vi "FXP info.vi"(8 "error in (no error)":errorcluster, 11 "Variant":variant) -> (0 "error out":errorcluster, 3 "child strings":string[](array[string]))   [LabVIEW 2019, in "DSF Configuration Utility.lvlib"]
uses:
  DSF Configuration Utility.lvlib
  <vilib>/Utility/Data Type/NI_Data Type.lvlib
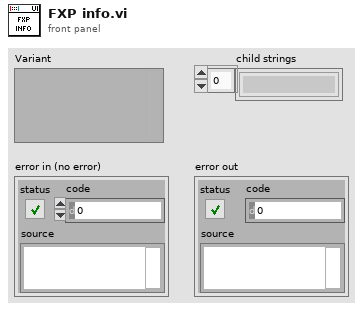
[diagram p1: front panel]
types:
  T1 = typedef "LVFixedPointRepRangeTypeDef.ctl" = cluster{"Range Min":dbl, "Range Max":dbl, "Delta":dbl}
  T2 = typedef "LVFixedPointRepBitsTypeDef.ctl" = cluster{"Signed":bool, "Word Length":u32, "Integer Word Length":i32}
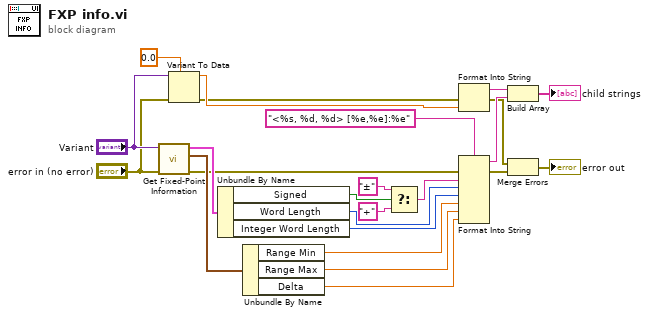
[diagram p0: block diagram]
diagram:
  n1 = call <vilib>:"Get Fixed-Point Information.vi"("error in (no error)"="error in (no error)", "variant"="Variant") -> ("error out"=w2:errorcluster, "FXP range"=w19:T1, "FXP representation"=w12:T2)  [unwired: 6 in, 1 out]
  n2 = Variant To Data(error in="error in (no error)", type=0.0, Variant="Variant") -> (data=w9:dbl, error out=w6:errorcluster)
  n3 = Unbundle By Name(w12) -> ("Signed"=w13:bool, "Word Length"=w17:u32, "Integer Word Length"=w18:i32)
  n4 = Unbundle By Name(w19) -> ("Range Min"=w20:dbl, "Range Max"=w21:dbl, "Delta"=w22:dbl)
  n5 = Select(t="±", s=w13, f="+" ("format string")) -> (s? t:f=w16:string)
  n6 = Format Into String(error in=w6, w9) -> (resulting string=w10:string, error out=w5:errorcluster)  [unwired: 2 in]
  n7 = Format Into String(format string="<%s, %d, %d> [%e,%e]:%e", error in=w2, w16, w17, w18, w20, w21, w22) -> (resulting string=w24:string, error out=w1:errorcluster)  [unwired: 1 in]
  n8 = Build Array(w10, w24) -> (→"child strings":string[])
  n9 = Merge Errors(w5, w1) -> (→"error out":errorcluster)
